vi "OpenSPI.vi"(8 "error in (no error)":errorcluster, 9 "Update Rate (4Hz-100Hz)":u8=100, 10 "Clock Rate (Hz)":dbl=2000000.0 format="%#_6f", 11 "SPI Bus":T1=enum."Invalid") -> (0 "error out":errorcluster, 3 "navX out":refnum<class "navX.lvclass">)   [LabVIEW 2015, in "navX Library v3.lvlib" / "navX.lvclass"]
uses:
  navX.lvclass
  <vilib>/Rock Robotics/SystemInterfaces/spilib/spi_bus.ctl
  navX - SPI/navX - SPI.lvclass
  navX - SPI/navX - SPI.lvclass/navX - SPI.ctl
  navX.lvclass/navX.ctl
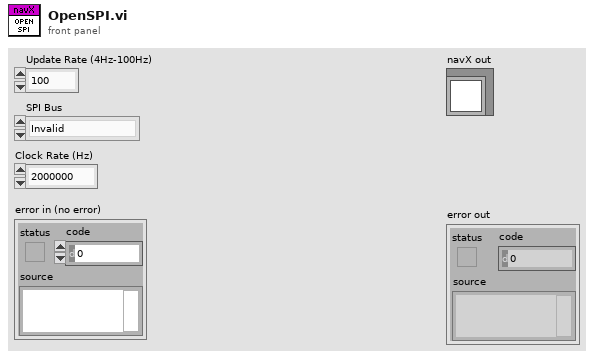
[diagram p1: front panel]
types:
  T1 = typedef "spi_bus.ctl" = enum16{"SPI On-Board, CS0", "SPI On-Board, CS1", "SPI On-Board, CS2", "SPI On-Board, CS3", "SPI MXP", "Invalid"}
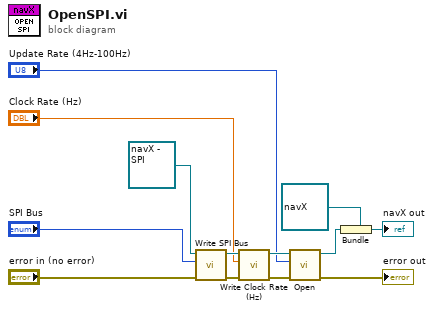
[diagram p0: block diagram]
diagram:
  n1 = call "Write SPI Bus.vi"("error in (no error)"="error in (no error)", "SPI Bus"="SPI Bus", "navX - SPI in"=refnum<class "navX - SPI.lvclass"> refnum ("navX Library v3.lvlib:navX - SPI.lvclass")) -> ("error out"=w9:errorcluster, "navX - SPI out"=w10:refnum<class "navX - SPI.lvclass">)  [unwired: 7 in]
  n2 = call "Write Clock Rate (Hz).vi"("error in (no error)"=w9, "Clock Rate (Hz)"="Clock Rate (Hz)", "navX - SPI in"=w10) -> ("error out"=w6:errorcluster, "navX - SPI out"=w7:refnum<class "navX - SPI.lvclass">)  [unwired: 7 in]
  n3 = call-dynamic "Open.vi"("error in (no error)"=w6, "Update Rate (4Hz-100Hz)"="Update Rate (4Hz-100Hz)", "navX - SPI in"=w7) -> ("error out"=→"error out":errorcluster, "navX - SPI out"=w3:refnum<class "navX - SPI.lvclass">)  [unwired: 7 in]
  n4 = Bundle(cluster=refnum<class "navX.lvclass"> refnum ("navX Library v3.lvlib:navX.lvclass"), w3) -> (→"navX out":refnum<class "navX.lvclass">)
